vi "Send Unregister Event.vi"(7 "Priority":T1=enum."Normal" caption="Message Priority (Normal)", 8 "error in (no error)":errorcluster, 9 "Registrant Address":refnum<class "Message Enqueuer.lvclass">, 10 "Event":refnum<class "Event.lvclass">, 11 "Message Enqueuer in":refnum<class "Message Enqueuer.lvclass">) -> (0 "error out":errorcluster, 3 "Message Enqueuer out":refnum<class "Message Enqueuer.lvclass">)   [LabVIEW 2016, in "Event Source.lvlib" / "Unregister Event Msg.lvclass"]
doc: "Sends the <b>Event Source.lvlib:Unregister Event Msg.lvclass</b> message.\n\nThis message will call <b>Unregister Event.vi</b> on the <b>Event Source.lvlib:Event Source.lvclass</b> actor.\n\n<b>Unregister Event.vi Description</b>\nThis method unregisters a specific Actors Enqueuer from specific Event he is listening to, in this Event Source Actor."
uses:
  Unregister Event Msg.lvclass
  <vilib>/ActorFramework/Message Enqueuer/Message Enqueuer.lvclass
  <vilib>/ActorFramework/Message Enqueuer/Message Priority.ctl
  Event/Event.lvclass
  C:/Program Files (x86)/National Instruments/LabVIEW 2016/vi.lib/ActorFramework/Message/Message.lvclass
  Unregister Event Msg.lvclass/Unregister Event Msg.ctl
  <vilib>/ActorFramework/Message Enqueuer/Message Enqueuer.lvclass/Message Enqueuer.ctl
  <vilib>/ActorFramework/Message Priority Queue/Priority Enqueue.vi
  <resource>/AFDebug/Generate Trace for Message.vi
  <vilib>/Utility/LVClass/Get LV Class Name.vi
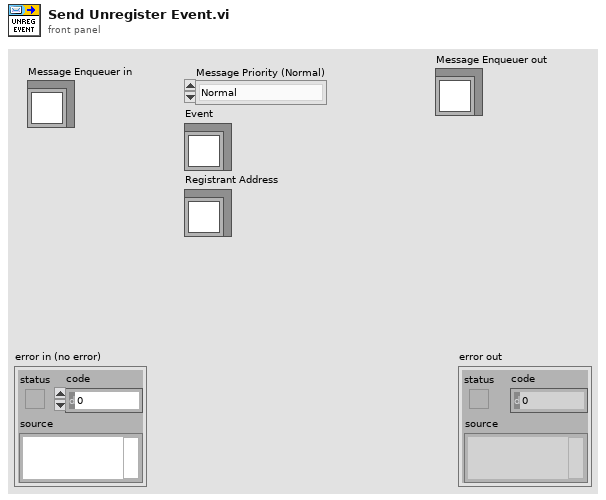
[diagram p1: front panel]
types:
  T1 = typedef "Actor Framework.lvlib/Message Enqueuer.lvclass/Message Priority.ctl" = enum16{"Low", "Normal", "High"}
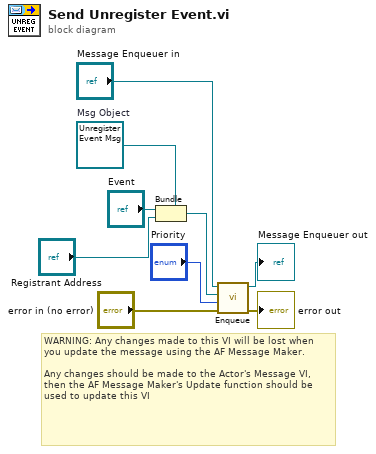
[diagram p0: block diagram]
diagram:
  w7 = refnum<class "Unregister Event Msg.lvclass"> refnum  # Msg Object
  # "WARNING: Any changes made to this VI will be lost when you update the message using the AF Message Maker.\n\nAny changes should be made to the Actor's Message VI, then the AF Message Maker's Update function should be used to update this VI"
  n1 = Bundle(cluster=w7, "Event", "Registrant Address") -> (w2:refnum<class "Unregister Event Msg.lvclass">)
  n2 = call <vilib>:"Enqueue.vi"("error in (no error)"="error in (no error)", "Message Priority (Normal)"="Priority", "Message"=w2, "Message Enqueuer in"="Message Enqueuer in") -> ("error out"=→"error out":errorcluster, "Message Enqueuer out"=→"Message Enqueuer out":refnum<class "Message Enqueuer.lvclass">)  [unwired: 6 in]
